vi "Calculate Min_Max FromTolerance.vi"(8 "error in":errorcluster, 10 "Tolerance(%)":dbl=10.0 format="%#_13g", 11 "Nominal Value":dbl=10.0 format="%#_13g") -> (0 "error out":errorcluster, 2 "MIN Limit":dbl, 3 "MAX Limit":dbl)   [LabVIEW 2023, in "HardwareAbstractionLayer_LVOOP.lvlib" / "Wait Monitor.lvclass"]
uses:
  Wait Monitor.lvclass
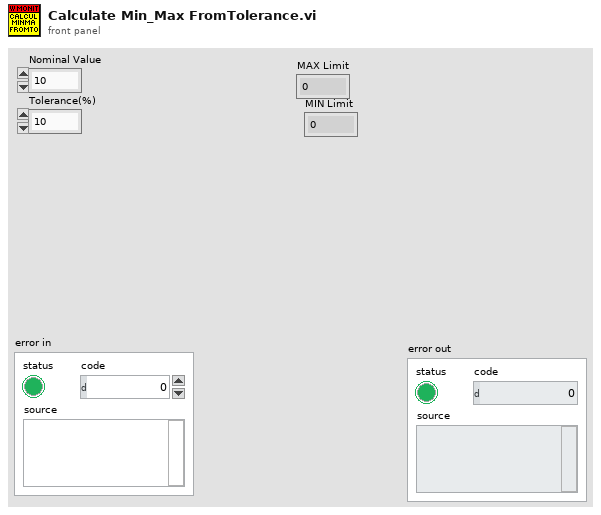
[diagram p1: front panel]
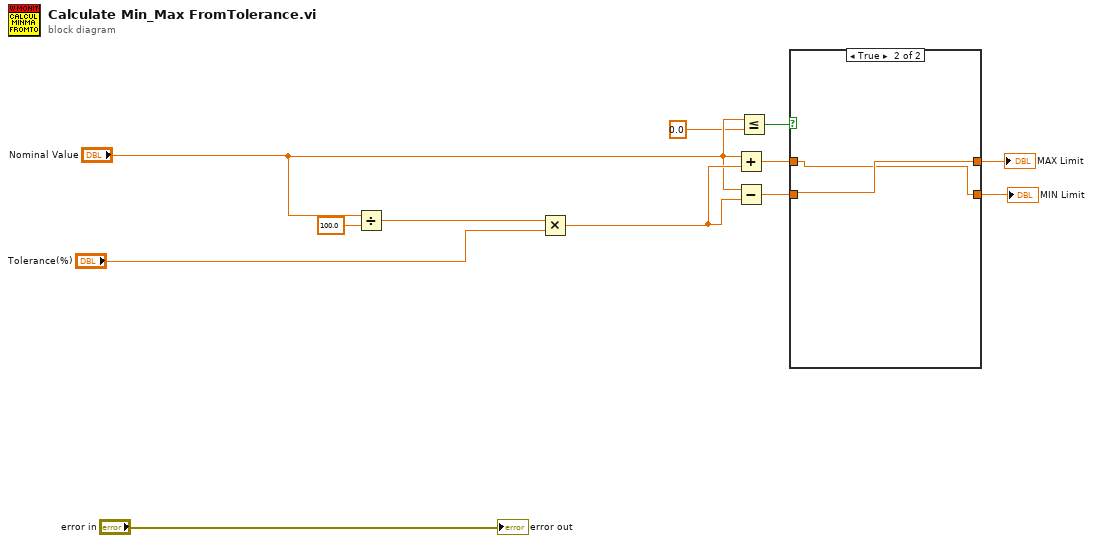
[diagram p0: block diagram]
diagram:
  n1 = Divide(x="Nominal Value", y=100.0) -> (x/y=w11:dbl)
  n2 = Multiply(x=w11, y="Tolerance(%)") -> (x*y=w9:dbl)
  n3 = Add(x="Nominal Value", y=w9) -> (x+y=w7:dbl)
  n4 = Subtract(x="Nominal Value", y=w9) -> (x-y=w5:dbl)
  n5 = Less Or Equal?(x="Nominal Value", y=0.0) -> (x <= y?=w2:bool)
  n6 = case shown="True" w2 {
    tunnel: w7 -> [w14 w15]
    tunnel: [w14 w16] -> w6
    tunnel: w5 -> [w13 w16]
    tunnel: [w13 w15] -> w4
    frame False {
    }
    frame True {
    }
  }
  "MAX Limit" <- w6
  "MIN Limit" <- w4
  "error out" <- "error in"
